vi "Leitura_Fluximetro.vi"() -> ()   [LabVIEW 2019]
panel:
  out "Vazão Mássica [kg/h]":dbl
  out "dt - Leitura Fluxímetro [s]":dbl
  out "Error Out":errorcluster
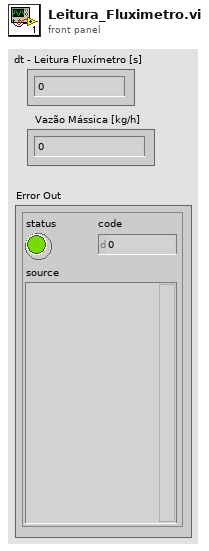
[diagram p1: front panel]
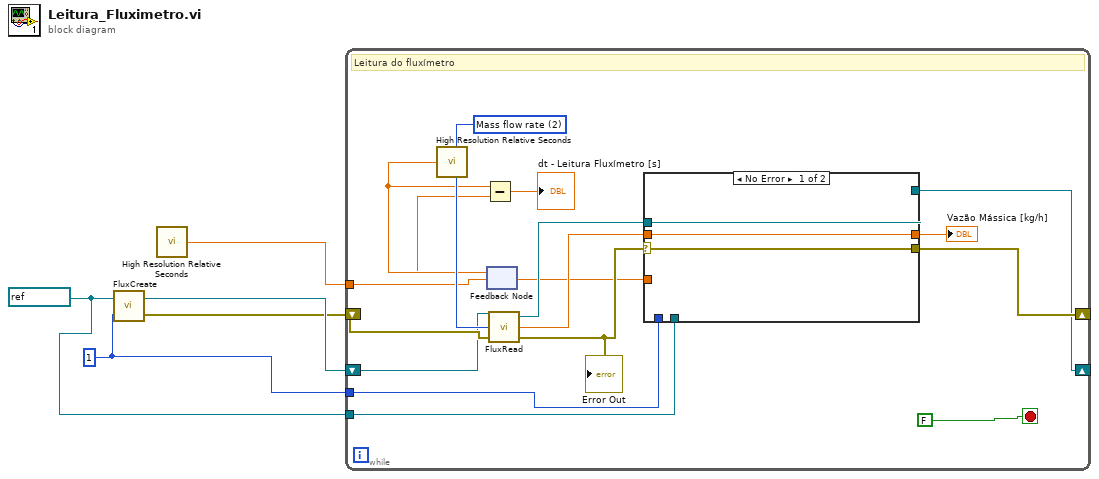
[diagram p0: block diagram]
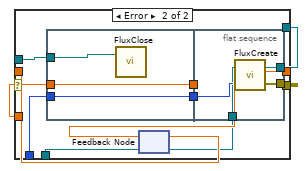
[diagram p2: hidden frame]
diagram:
  w2 = refnum<visa-resource-name> "COM3" ("VISA resource")
  w1 = u16 1 ("Endereço slave")
  n1 = call "FluxCreate.vi"("Endereço slave"=w1, "Recurso VISA"=w2) -> ("Error Out"=w3:errorcluster, "Master Out"=w4:refnum<class "Modbus Master.lvclass">)
  n2 = call <vilib>:"High Resolution Relative Seconds.vi"() -> ("relative seconds"=w5:dbl)
  n3 = while {
    tunnel: w5 -> [w12]
    tunnel: w2 -> [w7]
    tunnel: w1 -> [w10]
    shift-right: [w6] -> _
    shift-left: w4 -> [w9]
    shift-right: [w8] -> _
    shift-left: w3 -> [w11]
    stop <- FALSE stop-if-true
    w21 = 2 items=["Zero in progress", "Perform flowmeter zeroing", "Mass flow rate", "Density", "Temperature", "Volume flow rate", "Pressure (internally derived)", "Mass total", "Volume total", "Mass inventory", "Volume inventory", "Start/stop all totalizers", "Reset all totalizers", "Reset all inventories", "Real-time interrupt failure", "Sensor failure", "Temperature sensor failure", "Flowmeter zeroing failure", "Other failure occurred", "Mass flow rate meter factor", "Volume flow rate meter factor", "Density meter factor", "Flowing density calibration constant", "Mass flow scale factor", "Density scale factor", "Temperature scale factor", "Volume flow scale factor", "Pressure scale factor", "Mass total scale factor", "Volume total scale factor", "Mass inventory scale factor", "Volume inventory scale factor", "Flowmeter zeroing standard deviantion (units in microsec)", "Standard or special mass flow unit", "Density unit", "Temperature unit", "Standard or special volume flow unit", "Pressure unit", "Standard or special mass total or inventory unit", "Standard or special volume total or inventory unit", "Base mass unit for special mass unit", "Base time uni for special mass unit", "Base volume unit for special volume unit", "Base time unit for special volume unit", "Maximum zeroing time", "Flow direction", "EEProm checksum failure", "EEProm checksum failure in core processor", "EEProm database corrupt", "RAM diagnostic failure", "RAM diagnostic failure in core processor", "Real-time Interrupt failure", "Watchdog timer error", "Mass flow cutoff", "Volume flow cutoff", "Integer de erro 001", "Slug flow high-density limit (g/cm3)", "Slug flow low-density limit (g/cm3)"] ("Descrição da função leitura")
    # "Leitura do fluxímetro"
    n4 = call <vilib>:"High Resolution Relative Seconds.vi"() -> ("relative seconds"=w20:dbl)
    n5 = feedback #1() -> (w19:dbl)  [unwired: 1 in]
    n6 = Subtract(x=w20, y=w19) -> (x-y=→"dt - Leitura Fluxímetro [s]":dbl)
    n7 = feedback-in #1(w20) -> ()
    n8 = call "FluxRead.vi"("Error In"=w11, "Função de Leitura"=w21, "Master In"=w9) -> ("Error Out"=w14:errorcluster, "Data"=w16:dbl, "Master Out"=w17:refnum<class "Modbus Master.lvclass">)
    "Error Out" <- w14
    n9 = case shown="No Error" w14 {
      selector: w14 -> [w24 _]
      tunnel: w17 -> [w22 w30]
      tunnel: [w24 w33] -> w8
      tunnel: w12 -> [_ w34]
      tunnel: w16 -> [w23 w29]
      tunnel: [w23 w28] -> w15
      tunnel: w7 -> [_ w26]
      tunnel: w10 -> [_ w27]
      tunnel: [w22 w25] -> w6
      frame No Error {
      }
      frame Error {
        n10 = flat-sequence {
          tunnel: w34 -> [w36]
          tunnel: w27 -> [w37]
          tunnel: [w37] -> w32
          tunnel: [w36] -> w31
          tunnel: w30 -> [w35]
          tunnel: [w40] -> w33
          tunnel: w32 -> [w41]
          tunnel: w31 -> [_]
          tunnel: w26 -> [w39]
          tunnel: [w38] -> w25
          frame #0 {
            n11 = call "FluxClose.vi"("Master In"=w35) -> ()  [unwired: 1 in, 1 out]
          }
          frame #1 {
            n12 = call "FluxCreate.vi"("Endereço slave"=w41, "Recurso VISA"=w39) -> ("Error Out"=w40:errorcluster, "Master Out"=w38:refnum<class "Modbus Master.lvclass">)
          }
        }
        n13 = feedback-in #2(w29) -> ()
        n14 = feedback #2() -> (w28:dbl)  [unwired: 1 in]
      }
    }
    "Vazão Mássica [kg/h]" <- w15
  }
